vi "Framework Test.vi"() -> ()   [LabVIEW 2017]
uses:
  Classes/Framework/Framework.lvclass
  <vilib>/NI/Memory Manager/Classes/Pointer/Pointer.lvclass
  <vilib>/NI/Memory Manager/Classes/Pointer/Write Bool.vi
  Classes/Configuration Session/Configuration Session.lvclass
  Classes/Configuration/Framework/Framework Configuration.lvclass
  <vilib>/NI/Memory Manager/Classes/Pointer/Read Bool.vi
  <vilib>/NI/Memory Manager/Classes/Pointer/Write DBL.vi
  Typedefs/DSF Engine Framework Configuration.ctl
  DSF Core.lvlib
  Classes/Framework/Framework Options.ctl
  Typedefs/DSF Performance Options.ctl
  Typedefs/DSF FIFO Options.ctl
  Classes/Thread/Thread Options.ctl
  Classes/Thread/Thread.lvclass
  Typedefs/DSF Plugin Options.ctl
  Classes/Framework/Data Server Options.ctl
  Typedefs/DSF Timing Info.ctl
  Typedefs/DSF Settings Info.ctl
  Typedefs/DSF Engine Plugin Thread Configuration.ctl
  Typedefs/DSF Direction.ctl
  Typedefs/DSF Data Type.ctl
  Typedefs/DSF Engine Channel Configuration.ctl
  Typedefs/DSF Engine Transfer Configuration.ctl
  Typedefs/DSF Timeout Behavior.ctl
  Typedefs/DSF Engine Transfer Group Configuration.ctl
  Typedefs/DSF Engine Plugin Configuration.ctl
  Typedefs/DSF Version Info.ctl
  Typedefs/DSF Core Channel Configuration.ctl
  Typedefs/DSF Core Transfer Configuration.ctl
  Typedefs/DSF Core Group Configuration.ctl
  Typedefs/DSF Core Thread Configuration.ctl
  Typedefs/DSF Core Plugin Configuration.ctl
panel:
  in  "first channel":dbl format="%.3f"
  out "iteration":u64
  out "error out":errorcluster
  in  "framework options":T1={"FIFO Options"={"Infinite Timeouts"=FALSE}, "Thread Options"={"Show FP On Call"=TRUE, "Close FP After Call"=TRUE, "Allow Debugging"=TRUE}, "Plugin Options"={"Default Components"=TRUE}, "Performance Options"={"Measure Period"=TRUE, "Measure Rx/Tx Duration"=TRUE}, "Data Server Options"={"Enable Data Server"=TRUE, "Period"=50}} {"Data Server Options"."Period" format="%d ms"}
  in  "framework configuration":T7={"plugins"=[{"core"={"name"="Plugin", "components"=[], "cycle timing"={"priority"=10000, "decimation"=1, "offset"=0}}, "component settings"=[], "threads"=[]}]}
  in  "stop":bool
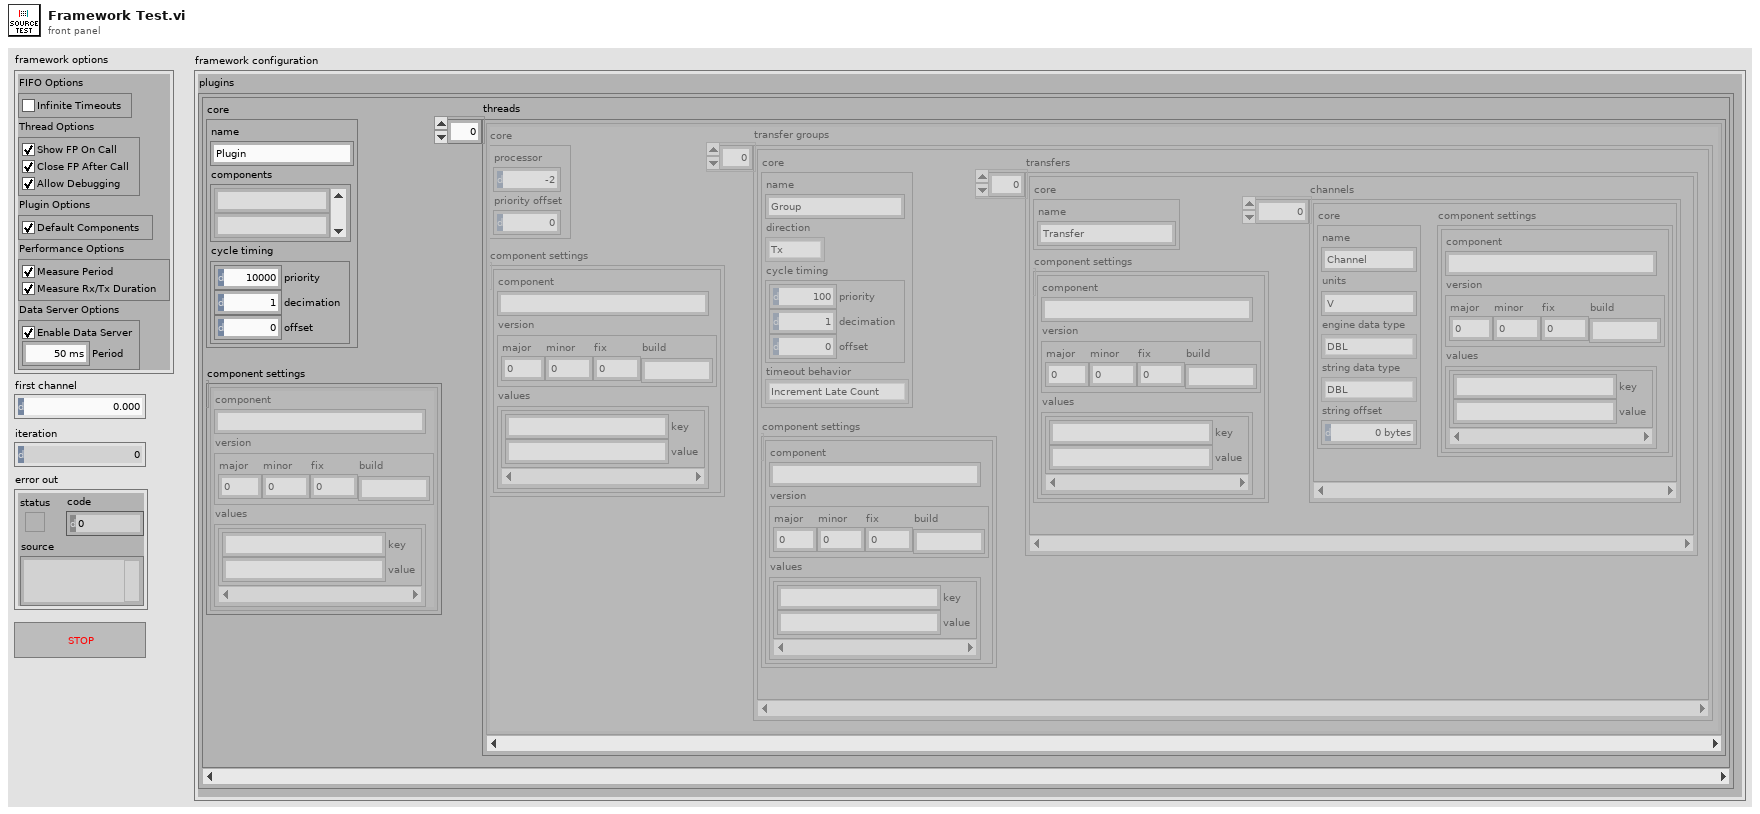
[diagram p1: front panel]
types:
  T1 = typedef "DSF Core.lvlib/Framework.lvclass/Framework Options.ctl" = cluster{"FIFO Options":T2, "Thread Options":T3, "Plugin Options":T4, "Performance Options":T5, "Data Server Options":T6}
  T2 = typedef "DSF Core.lvlib/Framework.lvclass/DSF FIFO Options.ctl" = cluster{"Infinite Timeouts":bool}
  T3 = typedef "DSF Core.lvlib/Thread.lvclass/Thread Options.ctl" = cluster{"Show FP On Call":bool, "Close FP After Call":bool, "Allow Debugging":bool}
  T4 = typedef "DSF Core.lvlib/Framework.lvclass/DSF Plugin Options.ctl" = cluster{"Default Components":bool}
  T5 = typedef "DSF Core.lvlib/DSF Performance Options.ctl" = cluster{"Measure Period":bool, "Measure Rx/Tx Duration":bool}
  T6 = typedef "DSF Core.lvlib/Framework.lvclass/Data Server Options.ctl" = cluster{"Enable Data Server":bool, "Period":u32}
  T7 = typedef "DSF Core.lvlib/DSF Engine Framework Configuration.ctl" = cluster{"plugins":T8[]}
  T8 = typedef "DSF Core.lvlib/DSF Engine Plugin Configuration.ctl" = cluster{"core":T9, "component settings":T11[], "threads":T13[]}
  T9 = typedef "DSF Core.lvlib/DSF Core Plugin Configuration.ctl" = cluster{"name":string, "components":string[], "cycle timing":T10}
  T10 = typedef "DSF Core.lvlib/DSF Timing Info.ctl" = cluster{"priority":u64, "decimation":u64, "offset":u64}
  T11 = typedef "DSF Core.lvlib/DSF Settings Info.ctl" = cluster{"component":string, "version":T12, "values":cluster{"key":string, "value":string}[]}
  T12 = typedef "DSF Core.lvlib/DSF Version Info.ctl" = cluster{"major":u32, "minor":u32, "fix":u32, "build":string}
  T13 = typedef "DSF Core.lvlib/DSF Engine Plugin Thread Configuration.ctl" = cluster{"core":T14, "component settings":T11[], "transfer groups":T15[]}
  T14 = typedef "DSF Core.lvlib/DSF Core Thread Configuration.ctl" = cluster{"processor":i32, "priority offset":i16}
  T15 = typedef "DSF Core.lvlib/DSF Engine Transfer Group Configuration.ctl" = cluster{"core":T16, "component settings":T11[], "transfers":T19[]}
  T16 = typedef "DSF Core.lvlib/DSF Core Group Configuration.ctl" = cluster{"name":string, "direction":T17, "cycle timing":T10, "timeout behavior":T18}
  T17 = typedef "DSF Core.lvlib/DSF Direction.ctl" = enum8{"Tx", "Rx"}
  T18 = typedef "DSF Core.lvlib/DSF Timeout Behavior.ctl" = enum8{"Increment Late Count", "Throw Error"}
  T19 = typedef "DSF Core.lvlib/DSF Engine Transfer Configuration.ctl" = cluster{"core":T20, "component settings":T11[], "channels":T21[]}
  T20 = typedef "DSF Core.lvlib/DSF Core Transfer Configuration.ctl" = cluster{"name":string}
  T21 = typedef "DSF Core.lvlib/DSF Engine Channel Configuration.ctl" = cluster{"core":T22, "component settings":T11[]}
  T22 = typedef "DSF Core.lvlib/DSF Core Channel Configuration.ctl" = cluster{"name":string, "units":string, "engine data type":T23, "string data type":T23, "string offset":u64}
  T23 = typedef "DSF Core.lvlib/DSF Data Type.ctl" = enum8{"Bool", "SGL", "DBL", "I8", "I16", "I32", "I64", "U8", "U16", "U32", "U64"}
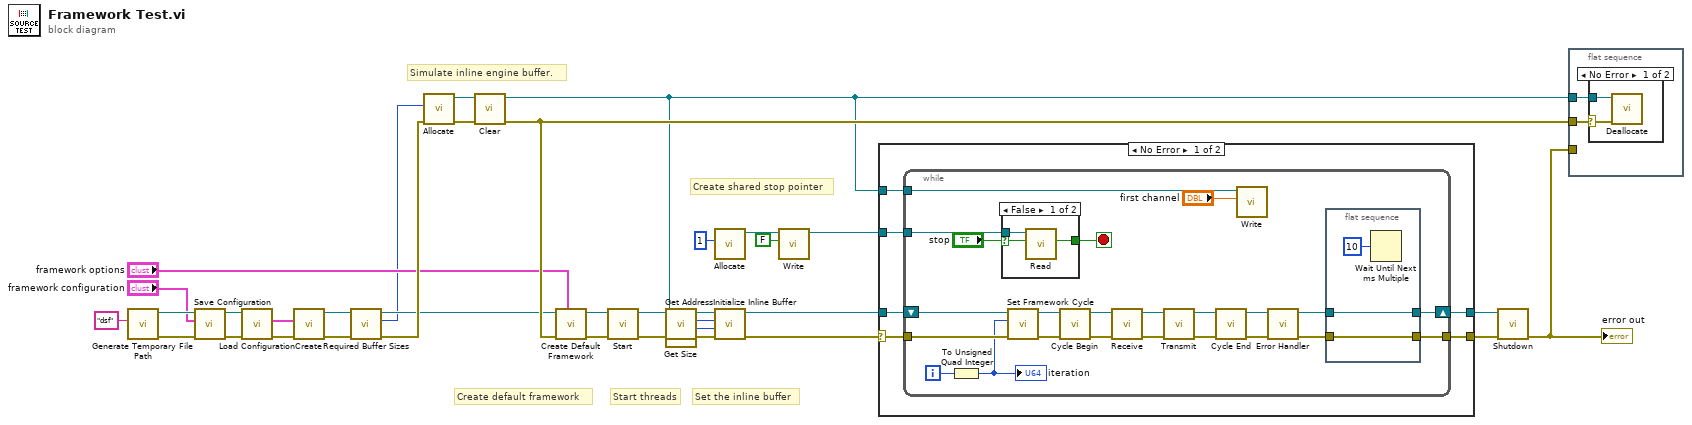
[diagram p0: block diagram]
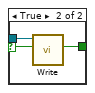
[diagram p3: hidden frame]
diagram:
  # "Create shared stop pointer"
  # "Set the inline buffer"
  # "Start threads"
  # "Create default framework"
  # "Simulate inline engine buffer."
  n1 = call <vilib>:"Generate Temporary File Path.vi"("Temporary File Extension (tmp)"="dsf") -> ("error out"=w11:errorcluster, "Unique Temporary File Path"=w14:path)  [unwired: 9 in]
  n2 = call "Save Configuration.vi"("error in (no error)"=w11, "configuration"="framework configuration", "configuration file path"=w14) -> ("error out"=w13:errorcluster, "configuration file path dup"=w12:path)  [unwired: 5 in, 2 out]
  n3 = call "Load Configuration.vi"("error in (no error)"=w13, "configuration file path"=w12) -> ("error out"=w8:errorcluster, "configuration"=w7:T7)  [unwired: 6 in, 2 out]
  n4 = call "Create.vi"("error in (no error)"=w8, "framework configuration"=w7) -> ("error out"=w6:errorcluster, "Framework Configuration out"=w5:refnum<class "Framework Configuration.lvclass">)  [unwired: 8 in]
  n5 = call-dynamic "Required Buffer Sizes.vi"("error in (no error)"=w6, "Framework Configuration in"=w5) -> ("error out"=w4:errorcluster, "engine size"=w1:u64, "Framework Configuration out"=w3:refnum<class "Framework Configuration.lvclass">)  [unwired: 6 in, 1 out]
  n6 = call <vilib>:"Allocate.vi"("error in (no error)"=w4, "size"=w1) -> ("error out"=w29:errorcluster, "Pointer out"=w26:refnum<class "Pointer.lvclass">)  [unwired: 8 in]
  n7 = call <vilib>:"Clear.vi"("error in (no error)"=w29, "Pointer in"=w26) -> ("error out"=w33:errorcluster, "Pointer out"=w9:refnum<class "Pointer.lvclass">)  [unwired: 8 in]
  n8 = call "Create Default Framework.vi"("framework options"="framework options", "error in (no error)"=w33, "Framework Configuration"=w3) -> ("error out"=w20:errorcluster, "Framework"=w25:refnum<class "Framework.lvclass">)  [unwired: 7 in]
  n9 = call-dynamic "Start.vi"("error in (no error)"=w20, "Framework in"=w25) -> ("error out"=w24:errorcluster, "Framework out"=w32:refnum<class "Framework.lvclass">)  [unwired: 8 in]
  n10 = call <vilib>:"Get Address.vi"("Pointer in"=w9) -> ("address"=w27:u64)  [unwired: 9 in, 1 out]
  n11 = call <vilib>:"Get Size.vi"("Pointer in"=w9) -> ("size"=w28:u64)  [unwired: 9 in, 1 out]
  n12 = call <vilib>:"Allocate.vi"("size"=u64 1) -> ("Pointer out"=w22:refnum<class "Pointer.lvclass">)  [unwired: 9 in, 1 out]
  n13 = call "Initialize Inline Buffer.vi"("error in (no error)"=w24, "size"=w28, "address"=w27, "Framework in"=w32) -> ("error out"=w18:errorcluster, "Framework out"=w16:refnum<class "Framework.lvclass">)  [unwired: 6 in]
  n14 = call-poly <vilib>:"Write.vi"("value"=FALSE, "Pointer in"=w22) -> ("Pointer out"=w17:refnum<class "Pointer.lvclass">)  [unwired: 6 in, 3 out]
  n15 = case shown="No Error" w18 {
    selector: w18 -> [w38 w72]
    tunnel: [w36 w72] -> w31
    tunnel: w16 -> [w39 w73]
    tunnel: [w37 w73] -> w30
    tunnel: w17 -> [w35 _]
    tunnel: w9 -> [w34 _]
    frame No Error {
      n16 = while {
        shift-right: [w60] -> w37
        shift-left: w39 -> [w54]
        tunnel: w35 -> [w57]
        tunnel: w38 -> [w53]
        tunnel: [w59] -> w36
        tunnel: w34 -> [w41]
        i -> [w58]
        stop <- w55 stop-if-true
        n17 = To Unsigned Quad Integer(1:w58) -> (0:w52:u64)
        "iteration" <- w52
        n18 = case shown="False" "stop" {
          selector: "stop" -> [w64 w67]
          tunnel: w57 -> [w65 w68]
          tunnel: [w63 w66] -> w55
          frame False {
            n19 = call-poly <vilib>:"Read.vi"("value in"=w64, "Pointer in"=w65) -> ("value out"=w63:bool)  [unwired: 6 in, 3 out]
          }
          frame True {
            n20 = call-poly <vilib>:"Write.vi"("value"=w67, "Pointer in"=w68) -> ("value"=w66:bool)  [unwired: 6 in, 3 out]
          }
        }
        n21 = call "Set Framework Cycle.vi"("error in (no error)"=w53, "iteration"=w52, "Framework in"=w54) -> ("error out"=w50:errorcluster, "Framework out"=w51:refnum<class "Framework.lvclass">)  [unwired: 7 in]
        n22 = call "Cycle Begin.vi"("error in (no error)"=w50, "Framework in"=w51) -> ("error out"=w48:errorcluster, "Framework out"=w49:refnum<class "Framework.lvclass">)  [unwired: 8 in]
        n23 = call "Receive.vi"("error in (no error)"=w48, "Framework in"=w49) -> ("error out"=w62:errorcluster, "Framework out"=w61:refnum<class "Framework.lvclass">)  [unwired: 8 in]
        n24 = call "Transmit.vi"("error in (no error)"=w62, "Framework in"=w61) -> ("error out"=w46:errorcluster, "Framework out"=w47:refnum<class "Framework.lvclass">)  [unwired: 8 in]
        n25 = call "Cycle End.vi"("error in (no error)"=w46, "Framework in"=w47) -> ("error out"=w44:errorcluster, "Framework out"=w45:refnum<class "Framework.lvclass">)  [unwired: 8 in]
        n26 = call-poly <vilib>:"Write.vi"("value"="first channel", "Pointer in"=w41) -> ()  [unwired: 6 in, 4 out]
        n27 = call "Error Handler.vi"("error in (no error)"=w44, "Framework in"=w45) -> ("error out"=w42:errorcluster, "Framework out"=w43:refnum<class "Framework.lvclass">)  [unwired: 8 in]
        n28 = flat-sequence {
          tunnel: w43 -> [w70]
          tunnel: w42 -> [w69]
          tunnel: [w70] -> w60
          tunnel: [w69] -> w59
          frame #0 {
            n29 = Wait Until Next ms Multiple(millisecond multiple=u32 10 ("milliseconds to wait")) -> ()  [unwired: 1 out]
          }
        }
      }
    }
    frame Error {
    }
  }
  n30 = call-dynamic "Shutdown.vi"("error in (no error)"=w31, "Framework in"=w30) -> ("error out"=w19:errorcluster)  [unwired: 8 in, 1 out]
  "error out" <- w19
  n31 = flat-sequence {
    tunnel: w9 -> [w75]
    tunnel: w19 -> [_]
    tunnel: w33 -> [w74]
    frame #0 {
      n32 = case shown="No Error" w74 {
        selector: w74 -> [w76 _]
        tunnel: w75 -> [w77 _]
        frame No Error {
          n33 = call <vilib>:"Deallocate.vi"("error in (no error)"=w76, "Pointer"=w77) -> ()  [unwired: 8 in, 2 out]
        }
        frame Error {
        }
      }
    }
  }
